vi "Load Bitfile Settings.vi"(8 "error in (no error)":errorcluster, 11 "bitfile path":path) -> (0 "error out":errorcluster, 1 "Bitfile Info":T1, 2 "Valid?":bool, 3 "SLSC version string":string)   [LabVIEW 2014, in "SLSC configuration System Explorer.lvlib"]
uses:
  SLSC configuration System Explorer.lvlib
  Type Defs/SLSC Bitfile Info.ctl
  Shared/Constants.vi
  Shared/SLSC configuration Shared.lvlib
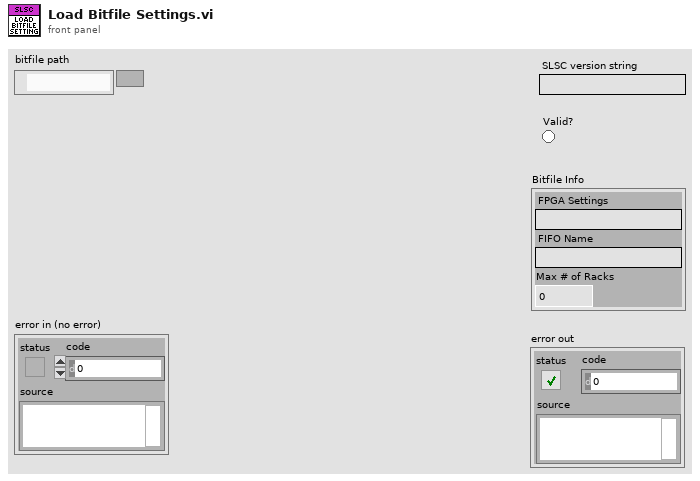
[diagram p1: front panel]
types:
  T1 = typedef "SLSC Bitfile Info.ctl" = cluster{"FPGA Settings":string, "FIFO Name":string, "Max # of Racks":i32}
  T2 = typedef "SLSC configuration System Explorer.lvlib/SLSC Custom Device Version.ctl" = enum8{"1.0"}
  T3 = typedef "niFpgaBitfileStructure_VI.ctl" = cluster{"Name":string, "RegisterMap":T4[], "Icon":T9}
  T4 = typedef "nirviControlStructure.ctl" = cluster{"Name":string, "Hidden":bool, "Indicator":bool, "Flattened Type":string, "Grouping":cluster{"Grouped":bool, "Member Names":string[], "Member IDs":u32[]}, "Address":u32, "Size":u32, "Class":u32, "Internal":bool, "Typedef":T5, "ID":u32, "Bidirectional":bool, "Synchronous":bool, "Mechanical Action":T6, "Sub Controls":T7[], "Access May Timeout":bool, "Register Node":bool}
  T5 = typedef "nirviTypdefDescription.ctl" = cluster{"Typedef":bool, "Path":path}
  T6 = typedef "nirviMechanicalAction.ctl" = enum8{"Switch When Pressed", "Switch When Released", "Switch Until Released", "Latch When Pressed", "Latch When Released", "Latch Until Released"}
  T7 = typedef "nirviSubControlStructure.ctl" = cluster{"Name":string, "flattened Type":string, "Cluster Information":T8, "Typedef":T5}
  T8 = typedef "nirviClusterElementControl.ctl" = cluster{"Name Hierarchy":string[], "Item Order":u32[]}
  T9 = typedef "imagedata.ctl" = cluster{"image type":i32, "image depth":i32, "image":u8[], "mask":u8[], "colors":u32[], "Rectangle":cluster{"left":i16, "top":i16, "right":i16, "bottom":i16}}
  T10 = typedef "SLSC configuration System Explorer.lvlib/Register Types.ctl" = enum16{"SLSC Settings", "# of Racks", "SPI FIFO Name"}
  T11 = cluster{"FPGA Settings":bool, "FIFO Name":bool, "Max # of Racks":bool}
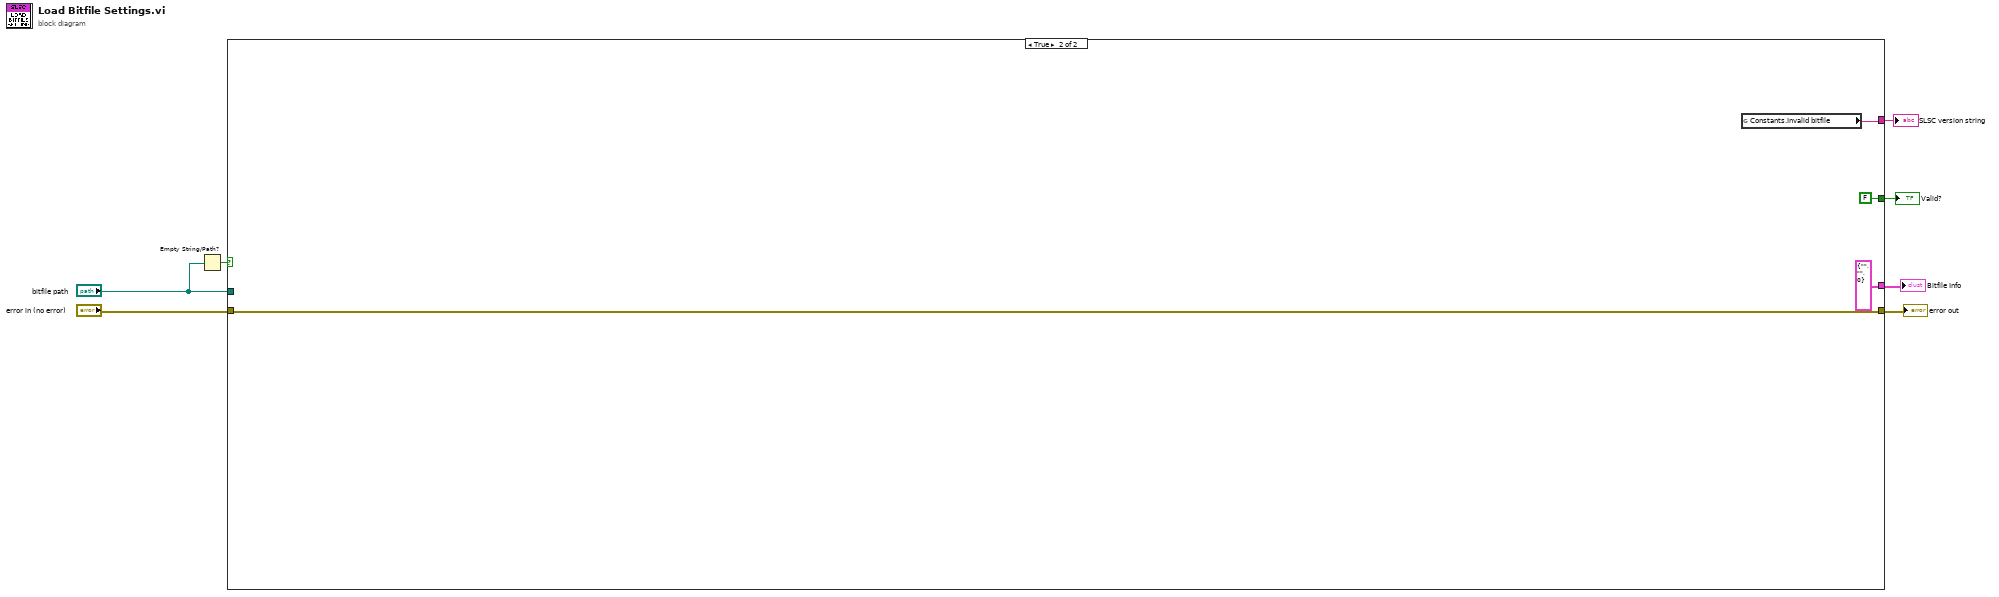
[diagram p0: block diagram]
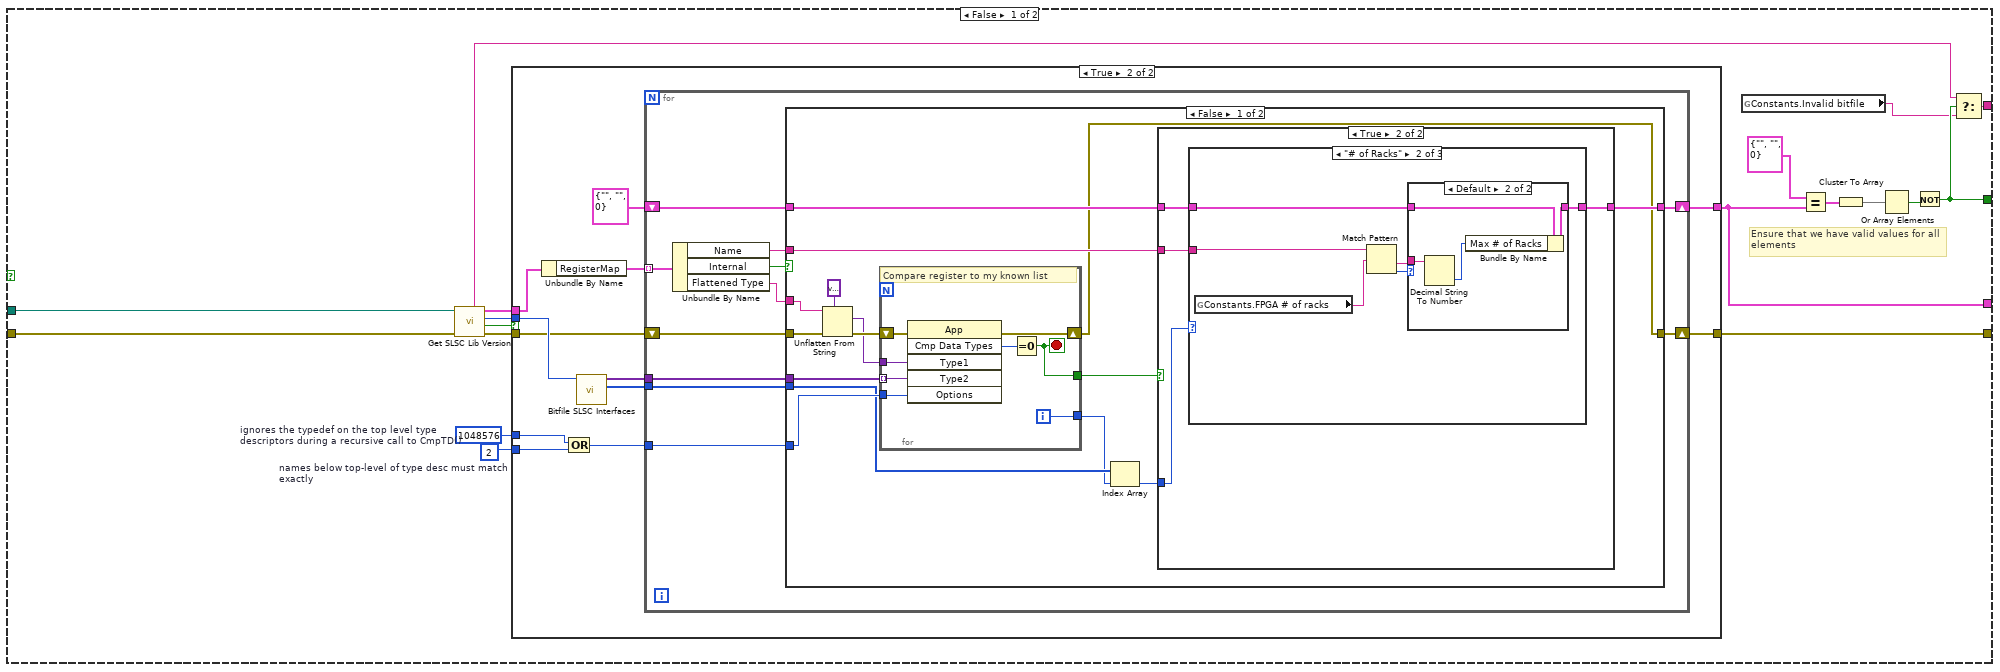
[diagram p2: hidden frame]
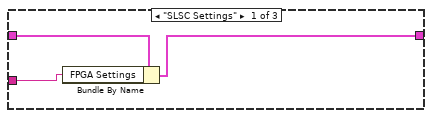
[diagram p5: hidden frame]
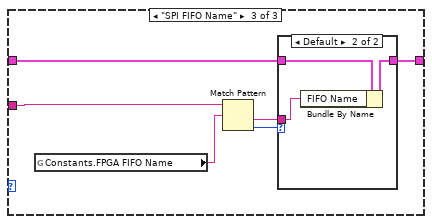
[diagram p7: hidden frame]
diagram:
  n1 = Empty String/Path?(string/path="bitfile path") -> (empty?=w1:bool)
  n2 = case shown="True" w1 {
    tunnel: [w18 T1 {"FPGA Settings"="", "FIFO Name"="", "Max # of Racks"=0} ("Cluster")] -> w7
    tunnel: "error in (no error)" -> [w14 w107]
    tunnel: [w13 w107] -> w5
    tunnel: [w12 FALSE] -> w4
    tunnel: [w9 w105] -> w3
    tunnel: "bitfile path" -> [w8 _]
    frame False {
      w20 = 2  # names below top-level of type desc must match exactly
      w21 = 1048576  # ignores the typedef on the top level type descriptors during a recursive call to CmpTD()
      # "Ensure that we have valid values for all\nelements"
      n3 = call "Get SLSC Lib Version.vi"("error in (no error)"=w14, "bitfile path"=w8) -> ("error out"=w22:errorcluster, "valid bitfile"=w25:bool, "SLSC version enum"=w24:T2, "vi info"=w23:T3, "SLSC version string"=w10:string)  [unwired: 5 in]
      n4 = case shown="True" w25 {
        tunnel: w24 -> [_ w38]
        tunnel: w23 -> [_ w37]
        tunnel: w22 -> [w26 w33]
        tunnel: w21 -> [_ w32]
        tunnel: w20 -> [_ w31]
        tunnel: [_ w28] -> w18
        tunnel: [w26 w27] -> w13
        frame False {
        }
        frame True {
          n5 = Unbundle By Name(w37) -> ("RegisterMap"=w36:T4[])
          n6 = Or(x=w32, y=w31) -> (x .or. y?=w30:i32)
          n7 = call "Bitfile SLSC Interfaces.vi"("SLSC CD Version"=w38) -> ("IP Types"=w34:T10[], "IP Interface"=w35:variant[])  [unwired: 9 in]
          n8 = for {
            tunnel: w36 -> [w49] mode=indexing
            tunnel: w35 -> [w45]
            tunnel: w34 -> [w44]
            tunnel: w30 -> [w43]
            shift-right: [w40] -> w28
            shift-left: T1 {"FPGA Settings"="", "FIFO Name"="", "Max # of Racks"=0} ("Cluster") -> [w42]
            shift-right: [w39] -> w27
            shift-left: w33 -> [w46]
            n9 = Unbundle By Name(w49) -> ("Name"=w41:string, "Internal"=w48:bool, "Flattened Type"=w47:string)
            n10 = case shown="False" w48 {
              tunnel: w47 -> [w61 _]
              tunnel: w46 -> [w60 w102]
              tunnel: w45 -> [w59 _]
              tunnel: w44 -> [w57 _]
              tunnel: w43 -> [w58 _]
              tunnel: w42 -> [w53 w103]
              tunnel: w41 -> [w52 _]
              tunnel: [w51 w103] -> w40
              tunnel: [w50 w102] -> w39
              frame False {
                n11 = Unflatten From String(type=variant ("Variant"), binary string=w61, error in (no error)=w60) -> (value=w62:variant, error out=w64:errorcluster)  [unwired: 3 out]
                n12 = for {
                  shift-right: [w100] -> w50
                  shift-left: w64 -> [w101]
                  tunnel: w62 -> [w98]
                  tunnel: w59 -> [w97] mode=indexing
                  tunnel: [w96] -> w55
                  tunnel: [w95] -> w56
                  tunnel: w58 -> [w94]
                  i -> [w95]
                  stop <- w96 stop-if-true
                  # "Compare register to my known list"
                  n13 = invoke class="App" method="Cmp Data Types"(error in=w101, "Type1"=w98, "Type2"=w97, "Options"=w94) -> (error out=w100:errorcluster, "Compare Data Types"=w99:i32)  [unwired: 2 in, 4 out]
                  n14 = Equal To 0?(x=w99) -> (x = 0?=w96:bool)
                }
                n15 = Index Array(array=w57, index=w56) -> (element=w54:T10)
                n16 = case shown="True" w55 {
                  tunnel: w54 -> [_ w69]
                  tunnel: w53 -> [w65 w68]
                  tunnel: w52 -> [_ w67]
                  tunnel: [w65 w66] -> w51
                  frame False {
                  }
                  frame True {
                    n17 = case shown="\"# of Racks\"" w69 {
                      tunnel: w68 -> [w72 w75 w89]
                      tunnel: w67 -> [w71 w74 w87]
                      tunnel: [w70 w76 w88] -> w66
                      frame "SLSC Settings" {
                        n18 = Bundle By Name(cluster=w72, "FPGA Settings"=w71) -> (w70:T1)
                      }
                      frame "# of Racks" {
                        n19 = global read "Constants.vi" "Constants.FPGA # of racks"() -> (w78:string)
                        n20 = Match Pattern(string=w74, regular expression=w78) -> (after substring=w73:string, offset past match=w77:i32)  [unwired: 1 in, 2 out]
                        n21 = case shown="Default" w77 {
                          tunnel: w75 -> [w79 w83]
                          tunnel: [w79 w82] -> w76
                          tunnel: w73 -> [_ w81]
                          frame -1 {
                          }
                          frame Default {
                            n22 = Decimal String To Number(string=w81) -> (number=w80:i32)  [unwired: 2 in, 1 out]
                            n23 = Bundle By Name(cluster=w83, "Max # of Racks"=w80) -> (w82:T1)
                          }
                        }
                      }
                      frame "SPI FIFO Name" {
                        n24 = global read "Constants.vi" "Constants.FPGA FIFO Name"() -> (w85:string)
                        n25 = Match Pattern(string=w87, regular expression=w85) -> (after substring=w86:string, offset past match=w84:i32)  [unwired: 1 in, 2 out]
                        n26 = case shown="Default" w84 {
                          tunnel: w89 -> [w90 w93]
                          tunnel: [w90 w92] -> w88
                          tunnel: w86 -> [_ w91]
                          frame -1 {
                          }
                          frame Default {
                            n27 = Bundle By Name(cluster=w93, "FIFO Name"=w91) -> (w92:T1)
                          }
                        }
                      }
                    }
                  }
                }
              }
              frame True {
              }
            }
          }
        }
      }
      n28 = global read "Constants.vi" "Constants.Invalid bitfile"() -> (w11:string)
      n29 = Equal?(x=T1 {"FPGA Settings"="", "FIFO Name"="", "Max # of Racks"=0} ("Cluster"), y=w18) -> (x = y?=w17:T11)
      n30 = Cluster To Array(cluster=w17) -> (array=w16:bool[])
      n31 = Or Array Elements(Boolean array=w16) -> (logical OR=w15:bool)
      n32 = Not(x=w15) -> (.not. x?=w12:bool)
      n33 = Select(t=w10, s=w12, f=w11) -> (s? t:f=w9:string)
    }
    frame True {
      n34 = global read "Constants.vi" "Constants.Invalid bitfile"() -> (w105:string)
    }
  }
  "SLSC version string" <- w3
  "Bitfile Info" <- w7
  "Valid?" <- w4
  "error out" <- w5
